vi "tm_setarea_wview.vi"(8 "error in (no error)":errorcluster, 10 "Sub Region":T1, 11 "Handle in":u32) -> (0 "error out":errorcluster, 3 "Handle out":u32)   [LabVIEW 2023]
uses:
  tmcamcon.dll
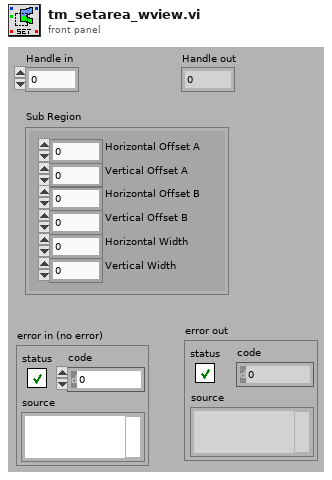
[diagram p1: front panel]
types:
  T1 = cluster{"Horizontal Offset A":i32, "Vertical Offset A":i32, "Horizontal Offset B":i32, "Vertical Offset B":i32, "Horizontal Width":i32, "Vertical Width":i32}
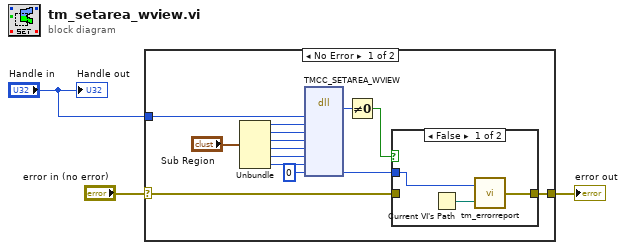
[diagram p0: block diagram]
diagram:
  n1 = case shown="No Error" "error in (no error)" {
    selector: "error in (no error)" -> [w15 w22]
    tunnel: [w12 w22] -> w2
    tunnel: "Handle in" -> [w16 _]
    frame No Error {
      n2 = Unbundle("Sub Region") -> ("Horizontal Offset A"=w10:i32, "Vertical Offset A"=w9:i32, "Horizontal Offset B"=w8:i32, "Vertical Offset B"=w7:i32, "Horizontal Width"=w6:i32, "Vertical Width"=w5:i32)
      n3 = dll-call lib="tmcamcon.dll" fn="TMCC_SETAREA_WVIEW"("HDCAM"=w16, "sho1"=w10, "svo1"=w9, "sho2"=w8, "svo2"=w7, "shw"=w6, "svw"=w5, "Erval"=0) -> ("return type"=w17:u32, "Erval"=w14:i32)  [unwired: 10 in, 2 out]
      n4 = Not Equal To 0?(x=w17) -> (x != 0?=w13:bool)
      n5 = case shown="False" w13 {
        tunnel: w15 -> [_ w21]
        tunnel: [w19 w21] -> w12
        tunnel: w14 -> [w18 _]
        frame False {
          n6 = Current VI's Path() -> (path=w20:path)
          n7 = call "tm_errorreport.vi"("Source"=w20, "Error"=w18) -> ("error out"=w19:errorcluster)
        }
        frame True {
        }
      }
    }
    frame Error {
    }
  }
  "error out" <- w2
  "Handle out" <- "Handle in"
